vi "test-numerical-jacobian-ab-callback-func.vi"(9 "U":T1, 10 "X":T1, 11 "Info":variant) -> (0 "Error":bool, 3 "XDOT":T1)   [LabVIEW 2019]
uses:
  <vilib>/Analysis/Matrix/Datatypes/RealMatrix.ctl
  <vilib>/Analysis/Matrix/NI_Matrix.lvlib
panel:
  in  "Cluster":cluster{"A":T1, "B":T1}
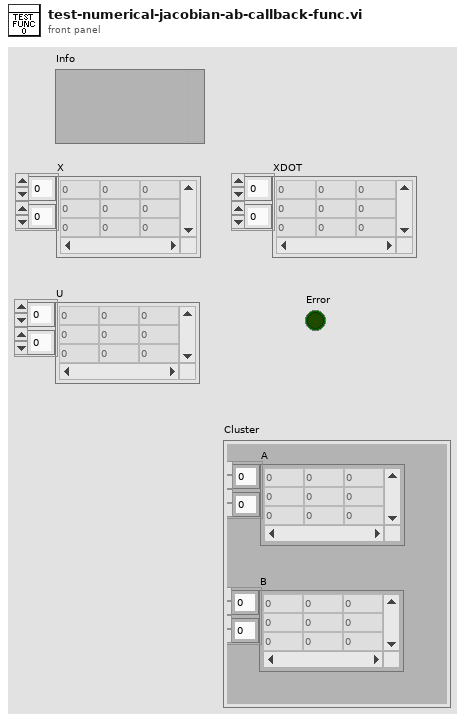
[diagram p1: front panel]
types:
  T1 = typedef "NI_Matrix.lvlib/RealMatrix.ctl" = dbl[][]
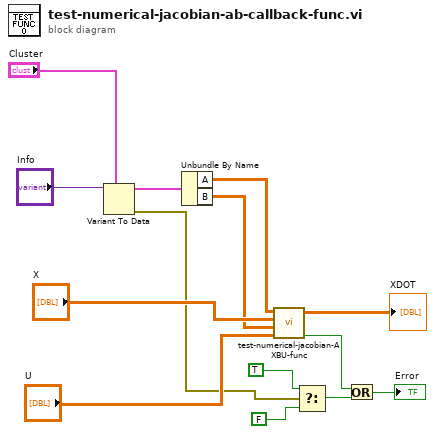
[diagram p0: block diagram]
diagram:
  n1 = Variant To Data(type="Cluster", Variant="Info") -> (data=w12:cluster{"A":T1, "B":T1}, error out=w1:errorcluster)  [unwired: 1 in]
  n2 = Unbundle By Name(w12) -> ("A"=w11:T1, "B"=w9:T1)
  n3 = call "test-numerical-jacobian-AXBU-func.vi"("U"="U", "B"=w9, "X"="X", "A"=w11) -> ("Error"=w5:bool, "OUT"=→"XDOT":T1)  [unwired: 6 in]
  n4 = Select(t=TRUE, s=w1, f=FALSE) -> (s? t:f=w4:bool)
  n5 = Or(x=w5, y=w4) -> (x .or. y?=→"Error":bool)
